vi "test_imu_3d.vi"() -> ()   [LabVIEW 2019]
uses:
  <vilib>/picture/3D Picture Control/NI_3D Picture Control.lvlib
  <vilib>/Instr/_visa.llb/VISA Configure Serial Port (Instr).vi
  <vilib>/picture/3D Picture Control/Object/Create Object (name).vi
  Ctrl/cmd_imu.ctl
panel:
  out "3D Picture":refnum<vi>(3d-picture)
  in  "Yaw":dbl(knob) scale=0.0..360.0
  in  "Roll":dbl(knob) scale=0.0..360.0
  in  "Pitch":dbl(knob) scale=0.0..360.0
  out "error out":errorcluster caption="에러 출력"
  in  "w":bool
  in  "w-data":string="ang"
  out "r buff":u32(graph)
  in  "baud rate":u32=115200 caption="rate"
  in  "Port":refnum<visa-resource-name>="COM24"
  in  "정지":bool
  out "Scene Display":refnum<vi>(3d-picture)
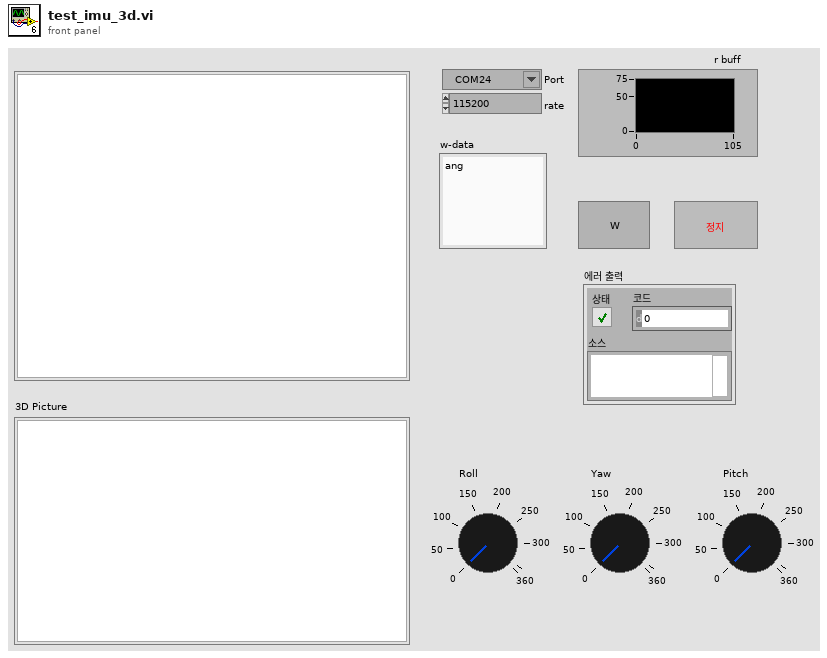
[diagram p1: front panel]
types:
  T1 = typedef "cmd_imu.ctl" = enum16{"ini", "write", "read"}
  T2 = cluster{"angle":dbl[], "acc":dbl[], "mag":dbl[], "gyr":dbl[]}
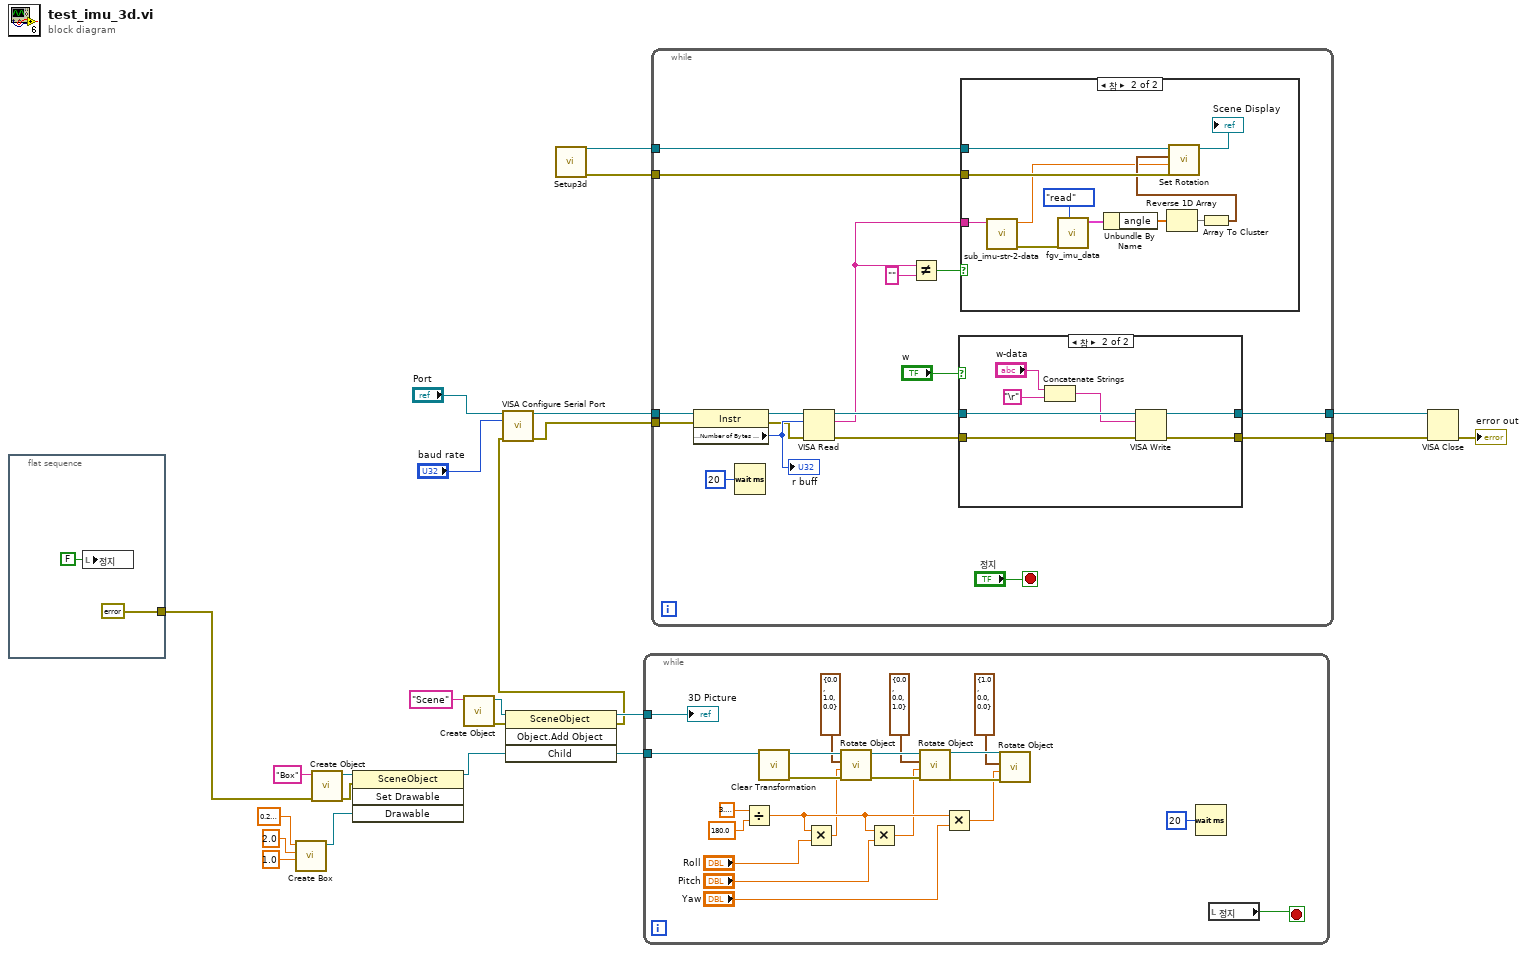
[diagram p0: block diagram]
diagram:
  n1 = flat-sequence {
    tunnel: [errorcluster {"status"=FALSE, "code"=0, "source"=""} ("error in (no error)")] -> w1
    frame #0 {
      n2 = local write "정지"(FALSE ("정지")) -> ()
    }
  }
  n3 = call <vilib>:"Create Box.vi"("Length Z"=sgl 1.0, "Length Y"=sgl 2.0, "Length X"=sgl 0.2) -> ("New Box Refnum"=w11:refnum<vi>)  [unwired: 7 in, 1 out]
  n4 = call-poly <vilib>:"Create Object.vi"("error in (no error)"=w1, "Name"="Box") -> ("error out"=w10:errorcluster, "Scene:New Object"=w9:refnum<vi>)  [unwired: 8 in]
  n5 = invoke class="SceneObject" method="Set Drawable"(reference=w9, error in=w10, "Drawable"=w11) -> (reference out=w15:refnum<vi>)  [unwired: 1 in, 3 out]
  n6 = call-poly <vilib>:"Create Object.vi"("Name"="Scene") -> ("error out"=w14:errorcluster, "Scene:New Object"=w13:refnum<vi>)  [unwired: 9 in]
  n7 = invoke class="SceneObject" method="Object.Add Object"(reference=w13, error in=w14, "Child"=w15) -> (reference out=w4:refnum<vi>, error out=w2:errorcluster, "Child"=w3:refnum<vi>)  [unwired: 1 in, 1 out]
  n8 = call-poly "VISA Configure Serial Port"("VISA resource name"="Port", "baud rate (9600)"="baud rate", "error in (no error)"=w2) -> ("VISA resource name out"=w19:refnum<visa-resource-name>, "error out"=w20:errorcluster)  [unwired: 11 in]
  n9 = call "Setup3d.vi"() -> ("error out"=w24:errorcluster, "Scene Object"=w23:refnum<vi>)  [unwired: 10 in]
  n10 = while {
    tunnel: w4 -> [w34]
    tunnel: w3 -> [w48]
    stop <- w28 stop-if-true
    n11 = Divide(x=3.141592653589793, y=180.0) -> (x/y=w36:dbl)
    n12 = call <vilib>:"Clear Transformation.vi"("Object Refnum In"=w48) -> ("error out"=w44:errorcluster, "Object Refnum Out"=w45:refnum<vi>)  [unwired: 9 in]
    n13 = Multiply(x=w36, y="Roll") -> (x*y=w33:dbl)
    n14 = call <vilib>:"Rotate Object.vi"("error in (no error)"=w44, "Angle"=w33, "Axis"=cluster{"X":sgl, "Y":sgl, "Z":sgl} {"X"=0.0, "Y"=1.0, "Z"=0.0}, "Scene.Object In"=w45) -> ("error out"=w46:errorcluster, "Scene.Object Out"=w47:refnum<vi>)  [unwired: 6 in]
    n15 = Multiply(x=w36, y="Pitch") -> (x*y=w32:dbl)
    n16 = call <vilib>:"Rotate Object.vi"("error in (no error)"=w46, "Angle"=w32, "Axis"=cluster{"X":sgl, "Y":sgl, "Z":sgl} {"X"=0.0, "Y"=0.0, "Z"=1.0}, "Scene.Object In"=w47) -> ("error out"=w39:errorcluster, "Scene.Object Out"=w40:refnum<vi>)  [unwired: 6 in]
    n17 = Multiply(x=w36, y="Yaw") -> (x*y=w35:dbl)
    n18 = call <vilib>:"Rotate Object.vi"("error in (no error)"=w39, "Angle"=w35, "Axis"=cluster{"X":sgl, "Y":sgl, "Z":sgl} {"X"=1.0, "Y"=0.0, "Z"=0.0}, "Scene.Object In"=w40) -> ()  [unwired: 6 in, 2 out]
    n19 = Wait (ms)(milliseconds to wait=u32 20 ("대기 시간 (ms)")) -> ()  [unwired: 1 out]
    n20 = local read "정지"() -> (w28:bool)
    "3D Picture" <- w34
  }
  n21 = while {
    tunnel: w24 -> [w50]
    tunnel: w23 -> [w49]
    tunnel: w20 -> [w60]
    tunnel: w19 -> [w59]
    tunnel: [w55] -> w17
    tunnel: [w54] -> w16
    stop <- "정지" stop-if-true
    n22 = property class="Instr"(reference=w59, error in=w60) -> (reference out=w64:refnum<visa-resource-name>, error out=w61:errorcluster, "Serial Settings:Number of Bytes at Serial Port"=w62:u32)
    "r buff" <- w62
    n23 = Wait (ms)(milliseconds to wait=u32 20 ("대기 시간 (ms)")) -> ()  [unwired: 1 out]
    n24 = VISA Read(VISA resource name=w64, byte count=w62, error in (no error)=w61) -> (VISA resource name out=w56:refnum<visa-resource-name>, read buffer=w51:string, error out=w57:errorcluster)  [unwired: 1 out]
    n25 = Not Equal?(x=w51, y="") -> (x != y?=w53:bool)
    n26 = case shown="참" "w" {
      tunnel: w56 -> [w78 w85]
      tunnel: [w78 w84] -> w55
      tunnel: w57 -> [w77 w83]
      tunnel: [w77 w82] -> w54
      frame False {
      }
      frame True {
        n27 = Concatenate Strings("w-data", "\r") -> (w79:string)
        n28 = VISA Write(VISA resource name=w85, write buffer=w79, error in (no error)=w83) -> (VISA resource name out=w84:refnum<visa-resource-name>, error out=w82:errorcluster)  [unwired: 1 out]
      }
    }
    n29 = case shown="참" w53 {
      tunnel: w51 -> [_ w76]
      tunnel: w50 -> [_ w74]
      tunnel: w49 -> [_ w73]
      frame False {
      }
      frame True {
        n30 = call "sub_imu-str-2-data.vi"("read buffer"=w76) -> ("error out"=w72:errorcluster, "yaw"=w68:dbl)  [unwired: 9 in]
        n31 = call "fgv_imu_data.vi"("cmd"=cmd_imu."read", "error in"=w72) -> ("IMD data out"=w71:T2)  [unwired: 6 in, 3 out]
        n32 = Unbundle By Name(w71) -> ("angle"=w70:dbl[])
        n33 = Reverse 1D Array(array=w70) -> (reversed array=w67:dbl[])
        n34 = Array To Cluster(array=w67) -> (cluster=w69:cluster{"[0]":dbl, "[1]":dbl, "[2]":dbl})
        n35 = call <vilib>:"Set Rotation.vi"("error in (no error)"=w74, "Angle"=w68, "Axis"=w69, "Scene Object"=w73) -> ("Rotated Scene Object"=→"Scene Display":refnum<vi>)  [unwired: 6 in, 1 out]
      }
    }
  }
  n36 = VISA Close(VISA resource name=w17, error in (no error)=w16) -> (error out=→"error out":errorcluster)
